vi "Temperature Warnings.vi"() -> ()   [LabVIEW 2015]
doc: "This VI is used to determine the string to output to the weather station based on the current temperature and limit settings.\n\nInputs: Current Temperature (DBL), Minimum Temperature (DBL), and Maximum Temperature (DBL).\nOutputs: Warning Text (string) and Warning? (Boolean)."
panel:
  out "error out":errorcluster
  in  "error in (no error)":errorcluster
  out "Warning Text":string="No Warning"
  out "Warning?":bool
  in  "Min Temperature":dbl
  in  "Max Temperature":dbl
  in  "Current Temperature":dbl
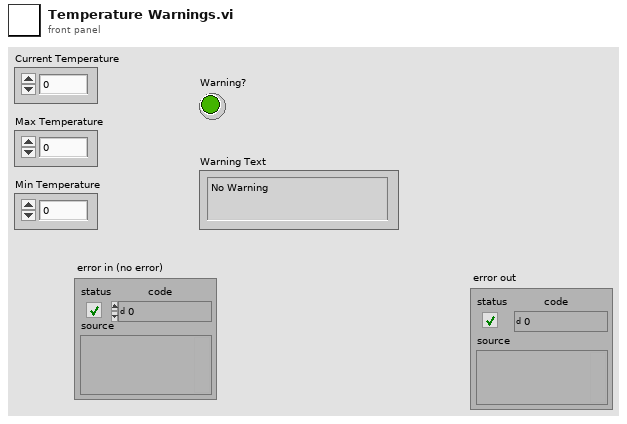
[diagram p1: front panel]
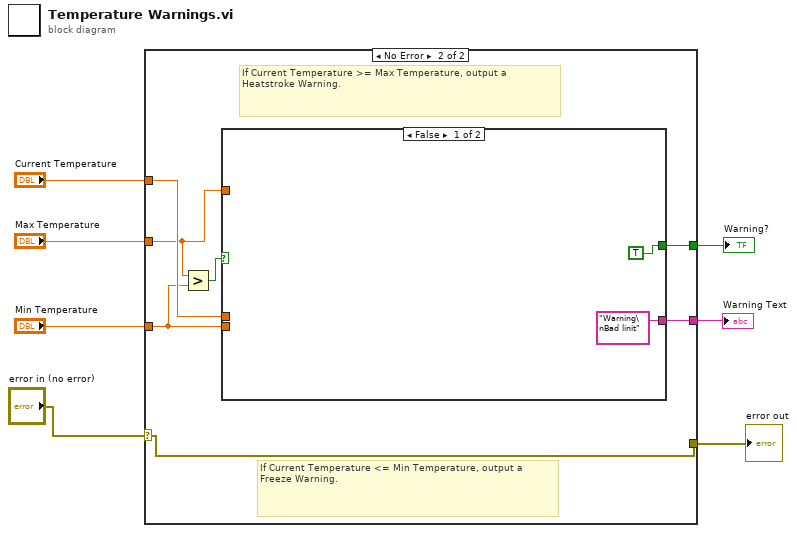
[diagram p0: block diagram]
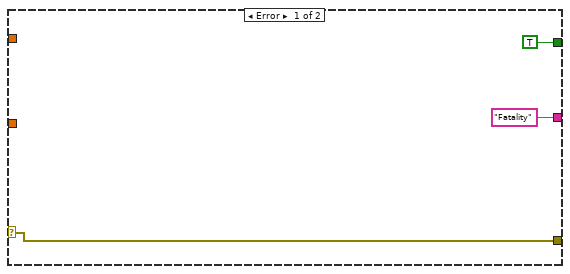
[diagram p2: hidden frame]
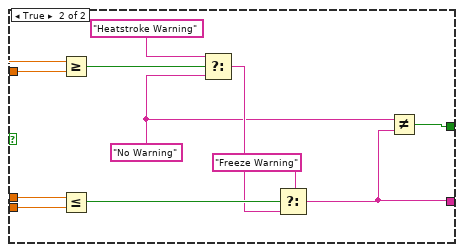
[diagram p3: hidden frame]
diagram:
  n1 = case shown="No Error" "error in (no error)" {
    selector: "error in (no error)" -> [w10 w14]
    tunnel: "Current Temperature" -> [_ w17]
    tunnel: "Min Temperature" -> [_ w12]
    tunnel: "Max Temperature" -> [_ w13]
    tunnel: [TRUE w16] -> w4
    tunnel: ["Fatality" ("f") w15] -> w3
    tunnel: [w10 w14] -> w1
    frame Error {
    }
    frame No Error {
      # "If Current Temperature >= Max Temperature, output a Heatstroke Warning."
      # "If Current Temperature <= Min Temperature, output a Freeze Warning."
      n2 = Greater?(x=w13, y=w12) -> (0:w11:bool)
      n3 = case shown="False" w11 {
        tunnel: w17 -> [_ w30]
        tunnel: w12 -> [_ w29]
        tunnel: w13 -> [_ w28]
        tunnel: [TRUE w27] -> w16
        tunnel: ["Warning\nBad linit" ("f") w26] -> w15
        frame False {
        }
        frame True {
          w20 = "No Warning" ("f")
          n4 = Greater Or Equal?(x=w30, y=w28) -> (x >= y?=w25:bool)
          n5 = Less Or Equal?(x=w30, y=w29) -> (x <= y?=w22:bool)
          n6 = Select(t="Heatstroke Warning", s=w25, f=w20) -> (s? t:f=w21:string)
          n7 = Select(t="Freeze Warning", s=w22, f=w21) -> (s? t:f=w26:string)
          n8 = Not Equal?(x=w20, y=w26) -> (x != y?=w27:bool)
        }
      }
    }
  }
  "Warning?" <- w4
  "Warning Text" <- w3
  "error out" <- w1
